vi "Num AI Ch to KH Ch Labels.vi"(8 "error in (no error)":errorcluster, 11 "Number of AI":i32) -> (0 "error out":errorcluster, 3 "KH Ch []":string[](array[string]))   [LabVIEW 2016, in "Control Experiment UI.lvclass"]
uses:
  Control Experiment UI.lvclass
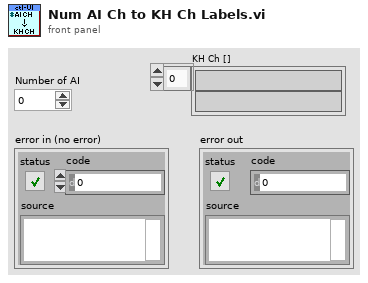
[diagram p1: front panel]
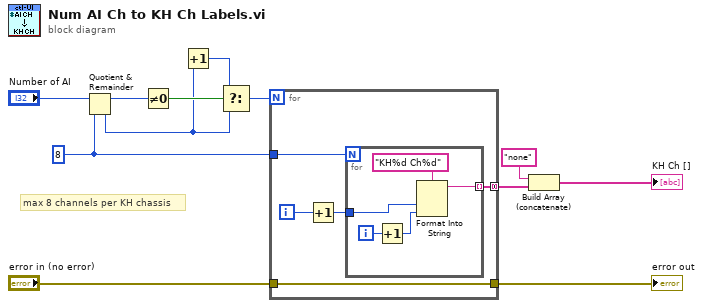
[diagram p0: block diagram]
diagram:
  w4 = 8 ("y")
  # "max 8 channels per KH chassis"
  n1 = Quotient & Remainder(x="Number of AI", y=w4) -> (x-y*floor(x/y)=w7:i32, floor(x/y)=w3:i32)
  n2 = Not Equal To 0?(x=w7) -> (x != 0?=w8:bool)
  n3 = Increment(x=w3) -> (x+1=w9:i32)
  n4 = Select(t=w9, s=w8, f=w3) -> (s? t:f=w10:i32)
  n5 = for {
    N: w10 -> [_]
    tunnel: [w17] -> w5 mode=concatenating
    tunnel: w4 -> [w16]
    tunnel: [w15] -> w12
    tunnel: "error in (no error)" -> [w15]
    i -> [w14]
    n6 = Increment(x=w14) -> (x+1=w13:i32)
    n7 = for {
      N: w16 -> [_]
      tunnel: w13 -> [w18]
      tunnel: [w20] -> w17 mode=indexing
      i -> [w21]
      n8 = Increment(x=w21) -> (x+1=w19:i32)
      n9 = Format Into String(format string="KH%d Ch%d", w18, w19) -> (resulting string=w20:string)  [unwired: 2 in, 1 out]
    }
  }
  "error out" <- w12
  n10 = Build Array (concatenate)("none", w5) -> (→"KH Ch []":string[])
